vi "create_cursor.vi"(8 "error in (no error)":errorcluster, 9 "x-location":dbl, 10 "operation":string(combo)="single cursor", 11 "XY Graph in":refnum<vi>) -> (0 "error out":errorcluster)   [LabVIEW 2017]
doc: "adds a cursor to the list of cursors\nor creates one single cursor for the plot.\nCursors are always vertical lines"
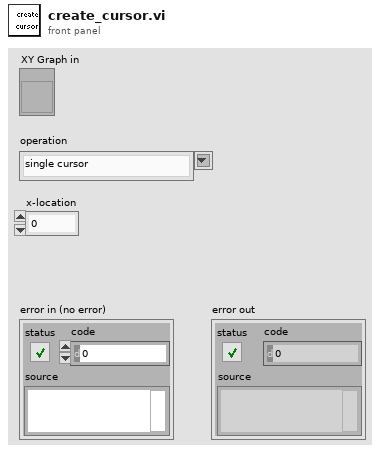
[diagram p1: front panel]
types:
  T1 = cluster{"Name":string, "Color":u32, "Style":u8, "Point Style":u8, "Name Visible":bool, "Allow Drag":bool, "Cursor Mode":u32, "Plot":i32, "Index":i32, "Position":cluster{"X":dbl, "Y":dbl}, "X Scale":u32, "Y Scale":u32, "Watch Plots":i32[], "Watch All Plots":bool, "Plot Area":i32, "Label Offset":cluster{"X":dbl, "Y":dbl}}
  T2 = typedef "LVCursorListTypeDef.ctl" = cluster{"Name":string, "Color":u32, "Style":u8, "Point Style":u8, "Name Visible":bool, "Allow Drag":bool, "Cursor Mode":u32, "Plot":i32, "Index":i32, "Position":cluster{"X":dbl, "Y":dbl}, "X Scale":u32, "Y Scale":u32, "Watch Plots":i32[], "Watch All Plots":bool, "Plot Area":i32, "Label Offset":cluster{"X":dbl, "Y":dbl}}[]
  T3 = cluster{"Name":string, "Color":u32, "Style":u8, "Point Style":u8, "Name Visible":bool, "Allow Drag":bool, "Cursor Mode":u32, "Plot":i32, "Index":i32, "Position":cluster{"X":dbl, "Y":dbl}, "X Scale":u32, "Y Scale":u32, "Watch Plots":i32[], "Watch All Plots":bool, "Plot Area":i32, "Label Offset":cluster{"X":dbl, "Y":dbl}}[]
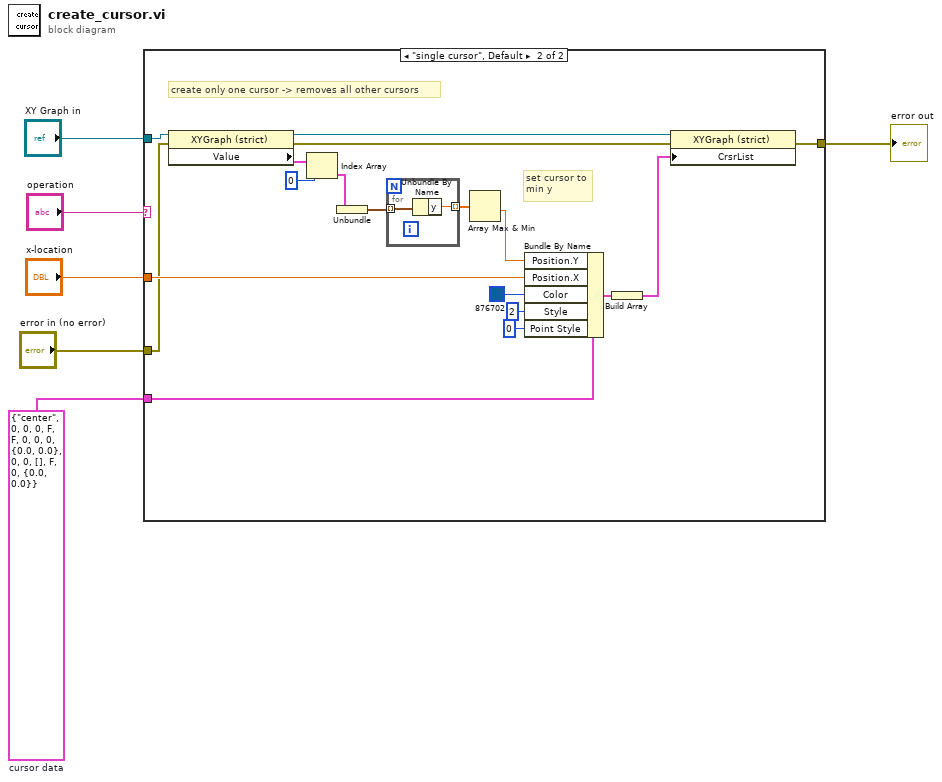
[diagram p0: block diagram]
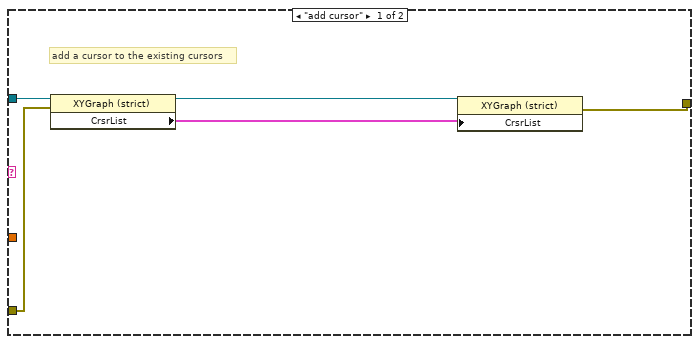
[diagram p2: hidden frame]
diagram:
  w3 = T1 {"Name"="center", "Color"=0, "Style"=0, "Point Style"=0, "Name Visible"=FALSE, "Allow Drag"=FALSE, "Cursor Mode"=0, "Plot"=0, "Index"=0, "Position"={"X"=0.0, "Y"=0.0}, "X Scale"=0, "Y Scale"=0, "Watch Plots"=[], "Watch All Plots"=FALSE, "Plot Area"=0, "Label Offset"={"X"=0.0, "Y"=0.0}}  # cursor data
  n1 = case shown="\"single cursor\", Default" "operation" {
    tunnel: "XY Graph in" -> [w11 w29]
    tunnel: "x-location" -> [_ w27]
    tunnel: "error in (no error)" -> [w10 w20]
    tunnel: w3 -> [_ w28]
    tunnel: [w9 w18] -> w2
    frame "add cursor" {
      # "add a cursor to the existing cursors"
      n2 = property class="XYGraph (strict)"(reference=w11, error in=w10) -> (reference out=w8:refnum<vi>, "CrsrList"=w7:T2)  [unwired: 1 out]
      n3 = property class="XYGraph (strict)"(reference=w8, "CrsrList"=w7) -> (error out=w9:errorcluster)  [unwired: 1 in, 1 out]
    }
    frame "single cursor", Default {
      # "set cursor to\nmin y"
      # "create only one cursor -> removes all other cursors"
      n4 = property on="Property Node" class="XYGraph (strict)"(reference=w29, error in=w20) -> (reference out=w26:refnum<vi>, error out=w19:errorcluster, "Value"=w15:cluster{cluster{"x":dbl, "y":dbl}[]}[])
      n5 = Index Array(array=w15, index=0) -> (element=w13:cluster{cluster{"x":dbl, "y":dbl}[]})
      n6 = Unbundle(w13) -> (w12:cluster{"x":dbl, "y":dbl}[])
      n7 = for {
        tunnel: w12 -> [w31] mode=indexing
        tunnel: [w30] -> w25 mode=indexing
        n8 = Unbundle By Name(w31) -> ("y"=w30:dbl)
      }
      n9 = Array Max & Min(array=w25) -> (min value=w24:dbl)  [unwired: 3 out]
      n10 = Bundle By Name(cluster=w28, "Position.Y"=w24, "Position.X"=w27, "Color"=u32 876702, "Style"=u8 2, "Point Style"=u8 0) -> (w22:T1)
      n11 = Build Array(w22) -> (w21:T3)
      n12 = property on="Property Node" class="XYGraph (strict)"(reference=w26, error in=w19, "CrsrList"=w21) -> (error out=w18:errorcluster)  [unwired: 1 out]
    }
  }
  "error out" <- w2
